vi "delta phase delta amp.vi"(9 "detection bar":dbl, 10 "signal in 2":waveform(dbl), 11 "signal in 1":waveform(dbl)) -> (1 "PSD 1":cluster{"f0":dbl, "df":dbl, "magnitude":dbl[]} {"magnitude" format="%.2p"; "f0" format="%0.2p"; "df" format="%0.2p"}, 2 "PSD 0":cluster{"f0":dbl, "df":dbl, "magnitude":dbl[]} {"magnitude" format="%.2p"; "f0" format="%0.2p"; "df" format="%0.2p"}, 3 "cal data":T1(array[cluster]))   [LabVIEW 2021]
uses:
  <vilib>/Analysis/4window.llb/windowTd.ctl
  <vilib>/Analysis/coordinate.llb/Angle Units.ctl
  <vilib>/Analysis/coordinate.llb/Angle Range (Degree).ctl
  <vilib>/Analysis/coordinate.llb/Wrap Angle (scalar).vi
  <vilib>/measure/maspectr.llb/FFT Spectrum (Mag-Phase) for 1 Chan.vi
  <vilib>/measure/NI_MAPro.lvlib
  <vilib>/Analysis/NI_AALPro.lvlib
  <vilib>/Analysis/NI_AAL_Angle.lvlib
  <vilib>/Analysis/NI_AAL_SigProc.lvlib
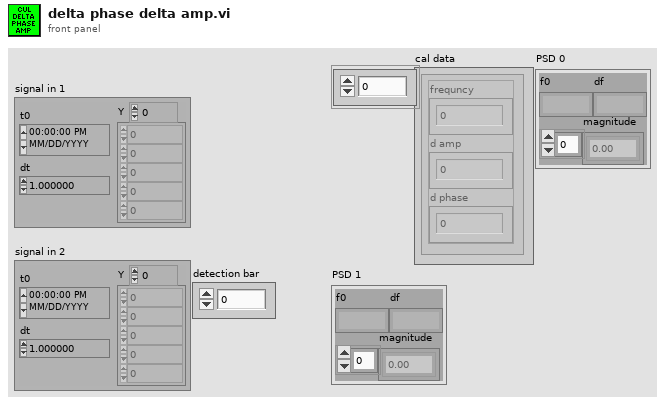
[diagram p1: front panel]
types:
  T1 = cluster{"frequncy":dbl, "d amp":dbl, "d phase":dbl}[]
  T2 = typedef "NI_AALPro.lvlib/windowTd.ctl" = u32
  T3 = cluster{"dB On (F)":bool, "unwrap phase (F)":bool, "convert to degree (F)":bool}
  T4 = cluster{"frequncy":dbl, "d amp":dbl, "d phase":dbl}
  T5 = typedef "NI_AAL_Angle.lvlib/Angle Range (Degree).ctl" = u16
  T6 = typedef "NI_AAL_Angle.lvlib/Angle Units.ctl" = i32
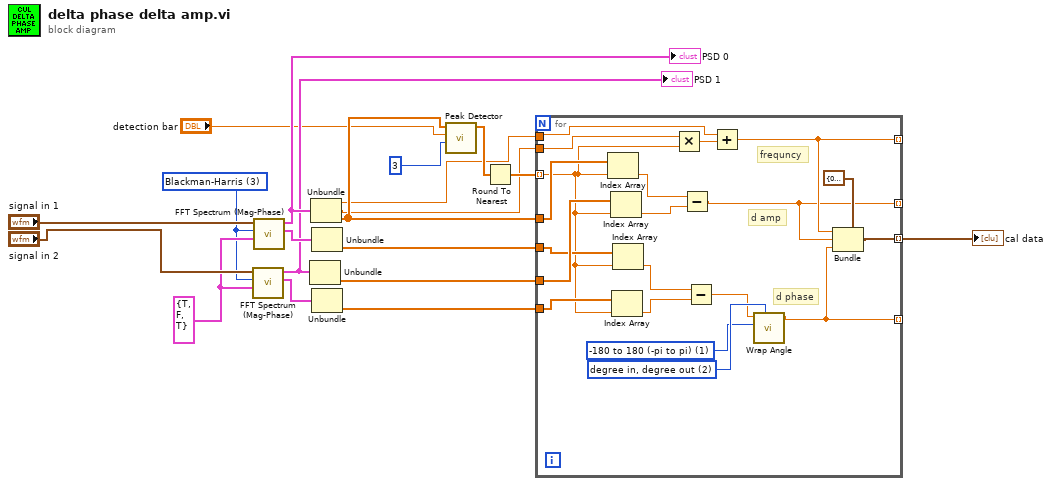
[diagram p0: block diagram]
diagram:
  w15 = T2 3 items=["Rectangle"=0, "Hanning"=1, "Hamming"=2, "Blackman-Harris"=3, "Exact Blackman"=4, "Blackman"=5, "Flat Top"=6, "4 Term B-Harris "=7, "7 Term B-Harris"=8, "Low Sidelobe"=9, "Blackman Nuttall"=11, "Triangle"=30, "Bartlett-Hanning"=31, "Bohman"=32, "Parzen"=33, "Welch"=34, "Kaiser"=60, "Dolph-Chebyshev"=61, "Gaussian"=62] ("window")
  w16 = T3 {"dB On (F)"=TRUE, "unwrap phase (F)"=FALSE, "convert to degree (F)"=TRUE} ("view")
  n1 = call-poly <vilib>:"FFT Spectrum (Mag-Phase).vi"("view"=w16, "window"=w15, "time signal"="signal in 2") -> ("phase"=w12:cluster{"f0":dbl, "df":dbl, "phase":dbl[]}, "magnitude"=w11:cluster{"f0":dbl, "df":dbl, "magnitude":dbl[]})  [unwired: 4 in, 3 out]
  "PSD 1" <- w11
  n2 = call-poly <vilib>:"FFT Spectrum (Mag-Phase).vi"("view"=w16, "window"=w15, "time signal"="signal in 1") -> ("phase"=w13:cluster{"f0":dbl, "df":dbl, "phase":dbl[]}, "magnitude"=w14:cluster{"f0":dbl, "df":dbl, "magnitude":dbl[]})  [unwired: 4 in, 3 out]
  "PSD 0" <- w14
  n3 = Unbundle(w11) -> ("magnitude"=w6:dbl[])  [unwired: 2 out]
  n4 = Unbundle(w14) -> ("f0"=w2:dbl, "df"=w3:dbl, "magnitude"=w8:dbl[])
  n5 = Unbundle(w13) -> ("phase"=w7:dbl[])  [unwired: 2 out]
  n6 = Unbundle(w12) -> ("phase"=w5:dbl[])  [unwired: 2 out]
  n7 = call <vilib>:"Peak Detector.vi"("width"=3, "threshold"="detection bar", "X"=w8) -> ("Locations"=w10:dbl[])  [unwired: 4 in, 4 out]
  n8 = Round To Nearest(number=w10) -> (nearest integer value=w9:dbl[])
  n9 = for {
    tunnel: w9 -> [w28] mode=indexing
    tunnel: w8 -> [w39]
    tunnel: w7 -> [w37]
    tunnel: w6 -> [w38]
    tunnel: w5 -> [w36]
    tunnel: [w21] -> _ mode=indexing
    tunnel: [w22] -> _ mode=indexing
    tunnel: w3 -> [w27]
    tunnel: w2 -> [w25]
    tunnel: [w23] -> _ mode=indexing
    tunnel: [w20] -> w1 mode=indexing
    w31 = T5 1 items=["none", "-180 to 180 (-pi to pi)", "0 to 360 (0 to 2pi)"] ("angle range")
    w33 = T6 2 items=["radian in, radian out", "radian in, degree out", "degree in, degree out", "degree in, radian out"] ("angle units")
    # "d phase"
    # "d amp"
    # "frequncy"
    n10 = Index Array(array=w39, index=w28) -> (element=w30:dbl)
    n11 = Index Array(array=w38, index=w28) -> (element=w29:dbl)
    n12 = Index Array(array=w36, index=w28) -> (element=w34:dbl)
    n13 = Index Array(array=w37, index=w28) -> (element=w35:dbl)
    n14 = Multiply(x=w27, y=w28) -> (x*y=w26:dbl)
    n15 = Subtract(x=w30, y=w29) -> (x-y=w22:dbl)
    n16 = Subtract(x=w35, y=w34) -> (x-y=w32:dbl)
    n17 = Add(x=w25, y=w26) -> (x+y=w23:dbl)
    n18 = call-poly <vilib>:"Wrap Angle.vi"("angle units"=w33, "angle range"=w31, "angle in"=w32) -> ("angle out"=w21:dbl)  [unwired: 7 in, 1 out]
    n19 = Bundle(cluster=T4 {"frequncy"=0.0, "d amp"=0.0, "d phase"=0.0}, "frequncy"=w23, "d amp"=w22, "d phase"=w21) -> (w20:T4)
  }
  "cal data" <- w1
